vi "State Check Digital Input 2.0.vi"(8 "Sys Error In":errorcluster, 10 "Step Description":string, 11 "Step Data String":string) -> (0 "Sys Error Out":errorcluster, 1 "Error No.":u16, 2 "Error String":string, 3 "Pass?":bool)   [LabVIEW 2018]
uses:
  05.UserVI's/type defs/EOL Global Digital Input Cluster Control.ctl
  05.UserVI's/type defs/EOL Global Digital Input Control.ctl
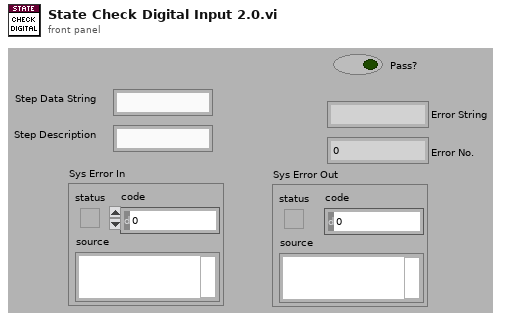
[diagram p1: front panel]
types:
  T1 = typedef "EOL Global Digital Input Cluster Control.ctl" = cluster{"EOL Global Digital Input Control":T2, "Input":bool}
  T2 = typedef "EOL Global Digital Input Control.ctl" = enum16{"Dev2/port0/line0", "Dev2/port0/line1", "Dev2/port0/line2", "Dev2/port0/line3", "Dev2/port0/line4", "Dev2/port0/line5", "Dev2/port0/line6", "Dev2/port0/line7", "Dev2/port1/line0", "Dev2/port1/line1", "Dev2/port1/line2", "Dev2/port1/line3", "Dev2/port1/line4", "Dev2/port1/line5", "Dev2/port1/line6", "Dev2/port1/line7", "Dev2/port2/line0", "Dev2/port2/line1", "Dev2/port2/line2", "Dev2/port2/line3", "Dev2/port2/line4", "Dev2/port2/line5", "Dev2/port2/line6", "Dev2/port2/line7", "Prerun Start Test", "Prerun Abort Test", "Audit Start Test", "Audit Abort Test", "Dev2/port3/line4", "Dev2/port3/line5", "Breakin Start Test", "Breakin Abort Test", "Not Implemented"}
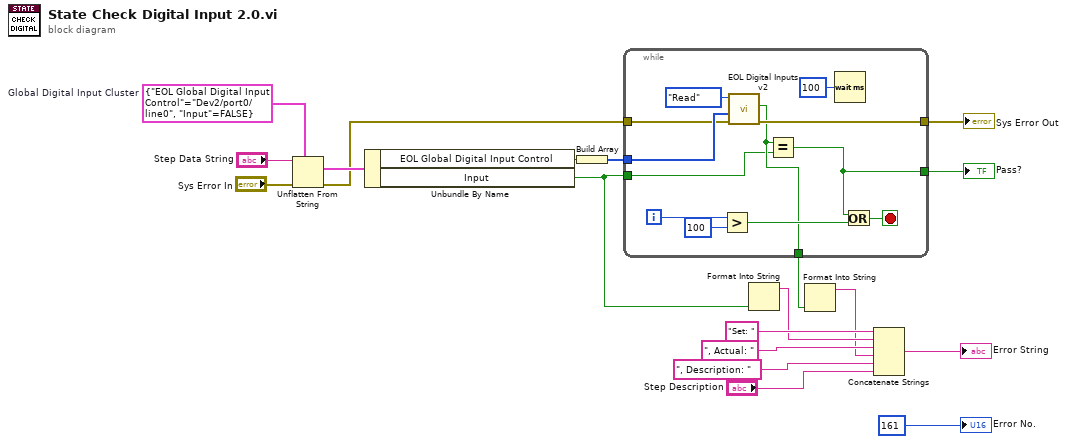
[diagram p0: block diagram]
diagram:
  w6 = T1 {"EOL Global Digital Input Control"=enum."Dev2/port0/line0", "Input"=FALSE}  # Global Digital Input Cluster
  n1 = Unflatten From String(type=w6, binary string="Step Data String", error in (no error)="Sys Error In") -> (value=w12:T1, error out=w2:errorcluster)  [unwired: 2 in, 1 out]
  n2 = Unbundle By Name(w12) -> ("EOL Global Digital Input Control"=w5:T2, "Input"=w9:bool)
  n3 = Build Array(w5) -> (w4:T2[])
  n4 = while {
    tunnel: [w20] -> w14
    tunnel: w9 -> [w21]
    tunnel: w4 -> [w30]
    tunnel: [w22] -> w3
    tunnel: w2 -> [w29]
    tunnel: [w28] -> w1
    i -> [w27]
    stop <- w25 stop-if-true
    n5 = Greater?(x=w27, y=100) -> (0:w24:bool)
    n6 = call "EOL Digital Inputs v2.vi"("Sys Error In"=w29, "Digital Inputs Array"=w30, "Mode"=enum16{"Init", "Read", "Read All", "Close"}."Read") -> ("Sys Error Out"=w28:errorcluster, "Single Input"=w22:bool)  [unwired: 6 in, 1 out]
    n7 = Equal?(x=w22, y=w21) -> (x = y?=w20:bool)
    n8 = Wait (ms)(milliseconds to wait=u32 100) -> ()  [unwired: 1 out]
    n9 = Or(x=w20, y=w24) -> (x .or. y?=w25:bool)
  }
  "Pass?" <- w14
  "Sys Error Out" <- w1
  n10 = Format Into String(w9) -> (resulting string=w8:string)  [unwired: 3 in, 1 out]
  n11 = Format Into String(w3) -> (resulting string=w7:string)  [unwired: 3 in, 1 out]
  n12 = Concatenate Strings("Set: " ("string"), w8, ", Actual: " ("string"), w7, ", Description: " ("string"), "Step Description") -> (→"Error String":string)
  "Error No." <- u8 161 ("Error No.")
